vi "ReplyCodeTesting.vi"() -> ()   [LabVIEW 2016]
panel:
  out "hello there 2":string
  out "hello there":string
  out "x33 x55 x77":string
  out "string 3":string="F"
  out "x33":string
  out "string":string="3"
  in  "Numeric":u8=51 format="%.0x"
  # "02 46 00 B9 C0 33 0C 02"
  # "Camera"
  # "185"
  # "12"
  # "192"
  # "Hub"
  # "b'\\x02F\\x00\\xb9\\xc03\\x0c\\x02'"
  # "hub.port.B.device.mode(0,b'\\x33')"
  # "b'\\x02F\\x00\\xb9\\xd03Uw\\x00>\\x02'"
  # "hub.port.B.device.mode(0,b'\\x33\\x55\\x77')"
  # "b'\\x02F\\x00\\xb9\\xe0\\\\hello there\\x00\\x00\\x00\\x00o\\x02'"
  # "hub.port.B.device.mode(0,b'\\hello there')"
  # "\\ = 5C = 92"
  # "b'\\x02F\\x00\\xb9\\xd0\n335577\n003E02"
  # "b'\\x02F\\x00\\xb9\\xd0\n3Uw\n\\x00>\\x02'"
  # "0 62 2"
  # "to do\nsend a Ctrl B when you close REPL"
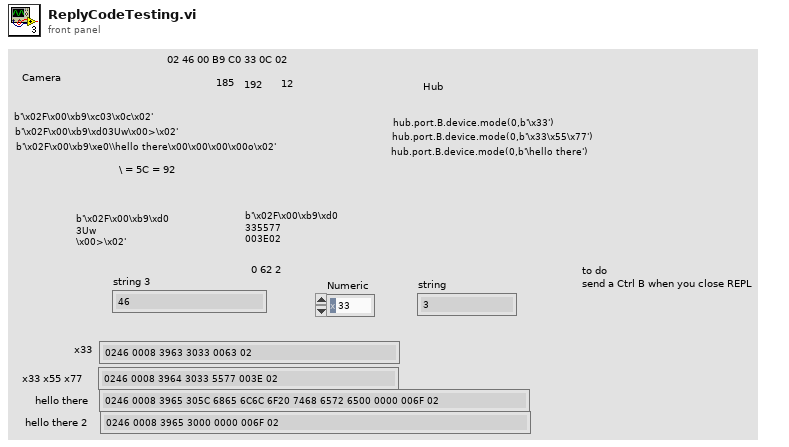
[diagram p1: front panel]
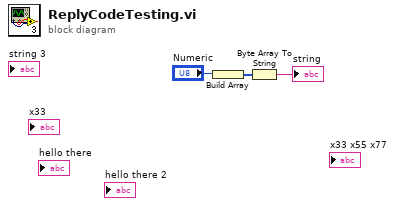
[diagram p0: block diagram]
diagram:
  n1 = Build Array("Numeric") -> (w2:u8[])
  n2 = Byte Array To String(unsigned byte array=w2) -> (string=→"string":string)
